vi "Write Bounds cluster ref.vi"(8 "error in (no error)":errorcluster, 10 "Bounds cluster":T1, 11 "Control-Client in":refnum<class "Control-Client.lvclass">) -> (0 "error out":errorcluster, 3 "Control-Client out":refnum<class "Control-Client.lvclass">)   [LabVIEW 2018, in "Control-Client.lvclass"]
uses:
  Control-Client.lvclass
  Control-Client.lvclass/Control-Client.ctl
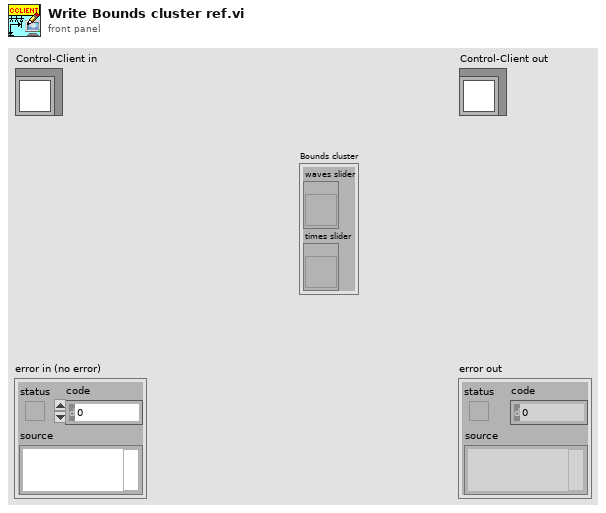
[diagram p1: front panel]
types:
  T1 = cluster{"waves slider":refnum<vi>, "times slider":refnum<vi>}
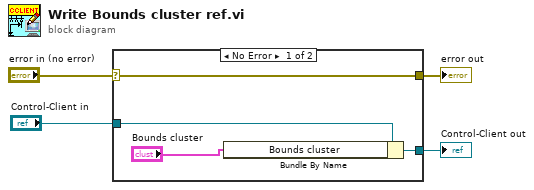
[diagram p0: block diagram]
diagram:
  n1 = case shown="No Error" "error in (no error)" {
    selector: "error in (no error)" -> [w8 w9]
    tunnel: [w8 w9] -> w3
    tunnel: [w6 w10] -> w1
    tunnel: "Control-Client in" -> [w7 w10]
    frame No Error {
      n2 = Bundle By Name(cluster=w7, "Bounds cluster"="Bounds cluster") -> (w6:refnum<class "Control-Client.lvclass">)
    }
    frame Error {
    }
  }
  "error out" <- w3
  "Control-Client out" <- w1
